vi "ComputeCenter from four straight edge lines.vi"(10 "Straight Edges top to bottom":T1(array[cluster]) {"Point2 (Real-World)"."Y" format="%.2f"; "Point2 (Real-World)"."X" format="%.2f"; "Point1 (Real-World)"."Y" format="%.2f"; "Point1 (Real-World)"."X" format="%.2f"; "Point2 (Pixels)"."Y" format="%.2f"; "Point2 (Pixels)"."X" format="%.2f"; "Point1 (Pixels)"."Y" format="%.2f"; "Point1 (Pixels)"."X" format="%.2f"}, 11 "Straight Edges Right to left":T1(array[cluster]) {"Point2 (Real-World)"."Y" format="%.2f"; "Point2 (Real-World)"."X" format="%.2f"; "Point1 (Real-World)"."Y" format="%.2f"; "Point1 (Real-World)"."X" format="%.2f"; "Point2 (Pixels)"."Y" format="%.2f"; "Point2 (Pixels)"."X" format="%.2f"; "Point1 (Pixels)"."Y" format="%.2f"; "Point1 (Pixels)"."X" format="%.2f"}) -> (3 "Solution Vector, y and x":dbl[](array[numeric]) format="%.2f")   [LabVIEW 2017]
doc: "Return an ordered pair, x and y, where the crosshair center is.\nBelieve it or not, there've been several crosshair edge calculations that are straight up and down.\nThe slope of the vertical crosshair is infinte, and the horizontal is 0. So there's a crappt case statement in there to handle the four cases, both have good slopes, both have 0 and inf slopes, and one or the other."
uses:
  <vilib>/Analysis/NI_AALPro.lvlib
  <vilib>/Analysis/7linalg.llb/Solve Linear Equations (single right hand).vi
  <vilib>/Analysis/Matrix/Datatypes/RealMatrix.ctl
  <vilib>/Analysis/Matrix/NI_Matrix.lvlib
panel:
  out "error":i32
  out "Solution Vector example":dbl[](array[numeric]) format="%.2f"
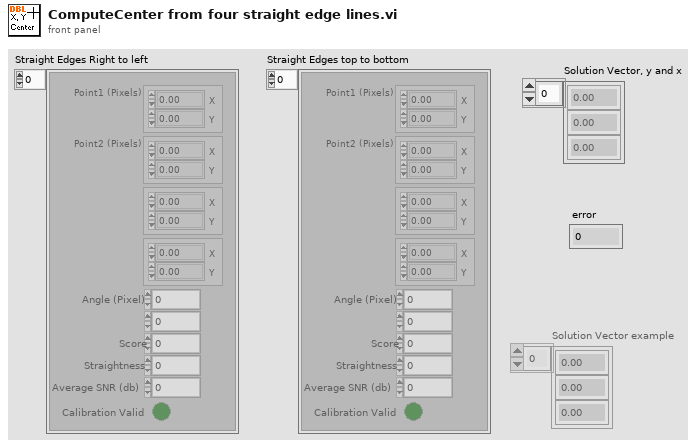
[diagram p1: front panel]
types:
  T1 = cluster{"Point1 (Pixels)":cluster{"X":sgl, "Y":sgl}, "Point2 (Pixels)":cluster{"X":sgl, "Y":sgl}, "Point1 (Real-World)":cluster{"X":sgl, "Y":sgl}, "Point2 (Real-World)":cluster{"X":sgl, "Y":sgl}, "Angle (Pixel)":dbl, "Angle (Real-World)":dbl, "Score":dbl, "Straightness":dbl, "Average SNR (db)":dbl, "Calibration Valid":bool}[]
  T2 = typedef "NI_Matrix.lvlib/RealMatrix.ctl" = dbl[][]
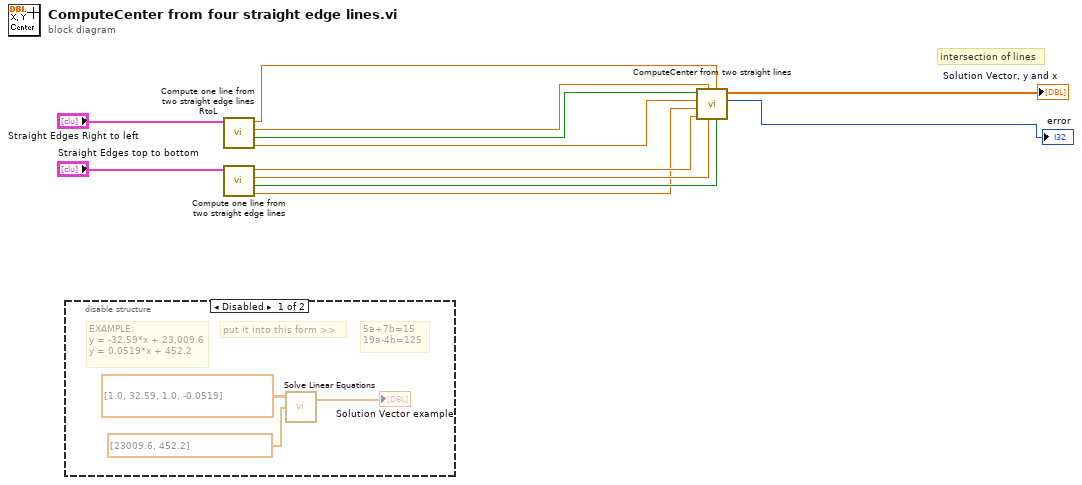
[diagram p0: block diagram]
diagram:
  # "intersection of lines"
  n1 = disable-structure shown="Disabled" {
    frame Disabled {
      # "put it into this form >>"
      # "EXAMPLE:\ny = -32.59*x + 23,009.6\ny = 0.0519*x + 452.2"
      # "5a+7b=15\n19a-4b=125"
      n2 = call-poly <vilib>:"Solve Linear Equations.vi"("Known Vector"=dbl[] [23009.6, 452.2], "Input Matrix"=T2 [[1.0, 32.59], [1.0, -0.0519]]) -> ("Solution Vector"=→"Solution Vector example":dbl[])  [unwired: 1 in, 1 out]
    }
    frame Enabled {
    }
  }
  n3 = call "Compute one line from two straight edge lines RtoL.vi"("Straight Edges"="Straight Edges Right to left") -> ("X"=w3:sgl, "x = 0?"=w7:bool, "intercept"=w6:dbl, "slope"=w9:dbl)  [unwired: 7 in]
  n4 = call "Compute one line from two straight edge lines.vi"("Straight Edges"="Straight Edges top to bottom") -> ("Y"=w1:sgl, "delta y = 0, slope 0"=w2:bool, "intercept"=w5:dbl, "slope"=w4:dbl)  [unwired: 7 in]
  n5 = call "ComputeCenter from two straight lines.vi"("delta y = 0, slope 0"=w2, "slope 2"=w9, "intercept"=w5, "intercept 2"=w6, "slope"=w4, "Y"=w1, "X"=w3, "x = 0?"=w7) -> ("error"=→"error":i32, "Solution Vector"=→"Solution Vector, y and x":dbl[])  [unwired: 2 in]
